vi "emi_Set Status Loop.vi"(5 "Loop ID in":u16, 7 "Running?":bool, 9 "error in (no error)":errorcluster) -> (6 "Loop ID out":u16, 10 "error out":errorcluster)   [LabVIEW 2011]
doc: "Input the execution state of the current loop"
uses:
  Private/_emi_Loop control int action.ctl
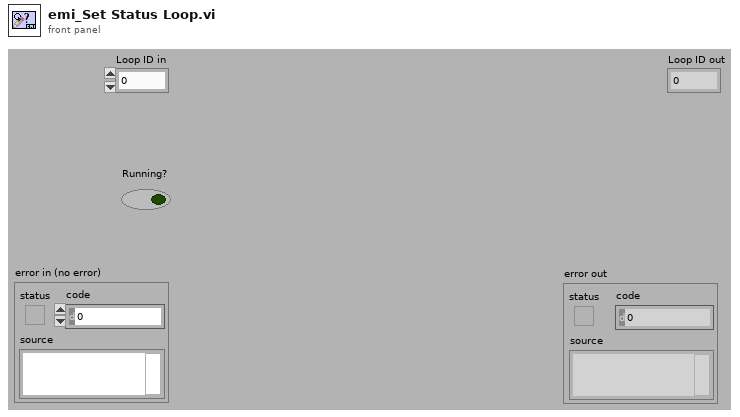
[diagram p1: front panel]
types:
  T1 = typedef "_emi_Loop control int action.ctl" = enum16{"Init index", "Get index", "Set index", "Get Size"}
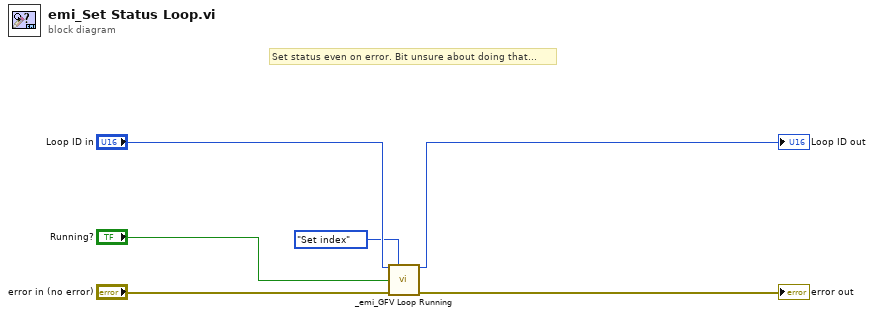
[diagram p0: block diagram]
diagram:
  # "Set status even on error. Bit unsure about doing that..."
  n1 = call "_emi_GFV Loop Running.vi"("Loop Index/Numb"="Loop ID in", "Action(Get Index)"=_emi_Loop_control_int_action."Set index", "Loop Running In(F)"="Running?", "error in (no error)"="error in (no error)") -> ("Index out"=→"Loop ID out":u16, "error out"=→"error out":errorcluster)  [unwired: 8 in, 2 out]
